vi "PZT read steps left.vi"(0 "VISA resource name":refnum<visa-resource-name> caption="VISA资源名称", 1 "error in (no error)":errorcluster caption="错误输入（无错误）") -> (2 "VISA资源名称输出":refnum<visa-resource-name>, 3 "Steps left":i32, 4 "错误输出":errorcluster)   [LabVIEW 2019]
uses:
  <vilib>/Utility/error.llb/DialogType.ctl
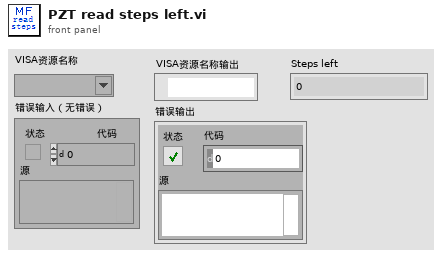
[diagram p1: front panel]
types:
  T1 = typedef "DialogType.ctl" = u16
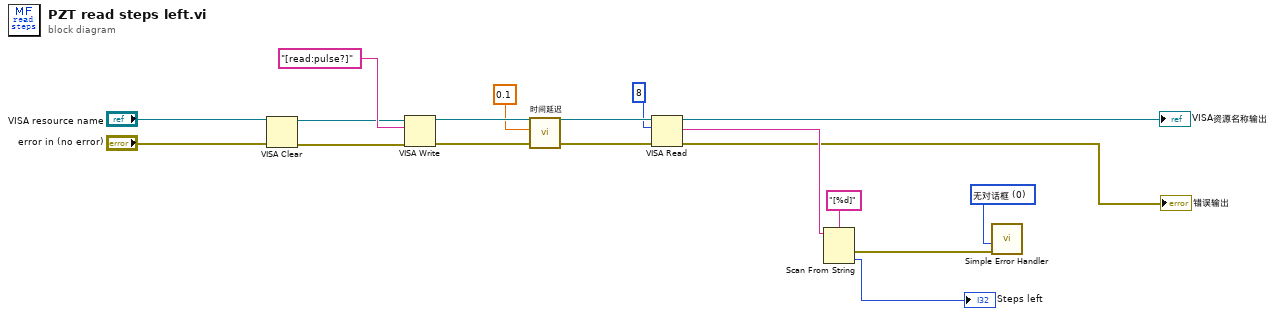
[diagram p0: block diagram]
diagram:
  w9 = T1 0 items=["无对话框", "确定信息", "继续或停止信息", "确定信息＋警告", "继续/停止+警告"] ("type of dialog (OK msg:1)")
  n1 = VISA Clear(VISA resource name="VISA resource name", error in (no error)="error in (no error)") -> (VISA resource name out=w4:refnum<visa-resource-name>, error out=w5:errorcluster)
  n2 = VISA Write(VISA resource name=w4, write buffer="[read:pulse?]" ("写入缓冲区"), error in (no error)=w5) -> (VISA resource name out=w15:refnum<visa-resource-name>, error out=w17:errorcluster)  [unwired: 1 out]
  n3 = call "时间延迟"("error in (no error)"=w17, "Delay Time (s)"=0.1) -> ("error out"=w16:errorcluster)  [unwired: 9 in]
  n4 = VISA Read(VISA resource name=w15, byte count=u32 8 ("字节总数"), error in (no error)=w16) -> (VISA resource name out=→"VISA资源名称输出":refnum<visa-resource-name>, read buffer=w12:string, error out=→"错误输出":errorcluster)  [unwired: 1 out]
  n5 = Scan From String(format string="[%d]" ("格式字符串"), input string=w12) -> (error out=w10:errorcluster, output 1=→"Steps left":i32)  [unwired: 3 in, 2 out]
  n6 = call <vilib>:"Simple Error Handler.vi"("type of dialog (OK msg:1)"=w9, "error in (no error)"=w10) -> ()  [unwired: 3 in, 5 out]
